vi "VT100translate.vi"(8 "cursor in":i32, 11 "Text":string) -> (0 "cursor out":i32, 3 "Console fixed":string)   [LabVIEW 2021]
panel:
  out "last \\n":i32
  out "string":string
  # "https://vt100.net/docs/vt100-ug/chapter3.html"
  # "http://braun-home.net/michael/info/misc/VT100_commands.htm"
  # "NoneLast login: Mon Aug  2 09:38:15 2021 from 127.0.0.1\n\n\n[1m[7m%[m[1m[0m                                                                               \n \n\n[0m[m[m[Jcrogers@Chriss-Pro ~ % [K[?2004h[?2004l\n\n[1m[7m%[m[1m[0m                                                                               \n \n\n[0m[m[m[Jcrogers@Chriss-Pro ~ % [K[?2004h[?2004l\n\n[1m[7m%[m[1m[0m                                                                               \n \n\n[0m[m[m[Jcrogers@Chriss-Pro ~ % [K[?2004h[?2004l\n\n[1m[7m%[m[1m[0m                                                                               \n \n\n[0m[m[m[Jcrogers@Chriss-Pro ~ % [K[?2004h?2004l\ncrogers@Chriss-Pro ~ % ?2004h?2004l\ncrogers@Chriss-Pro ~ % ?2004h"
  # "ESC [ 13D"
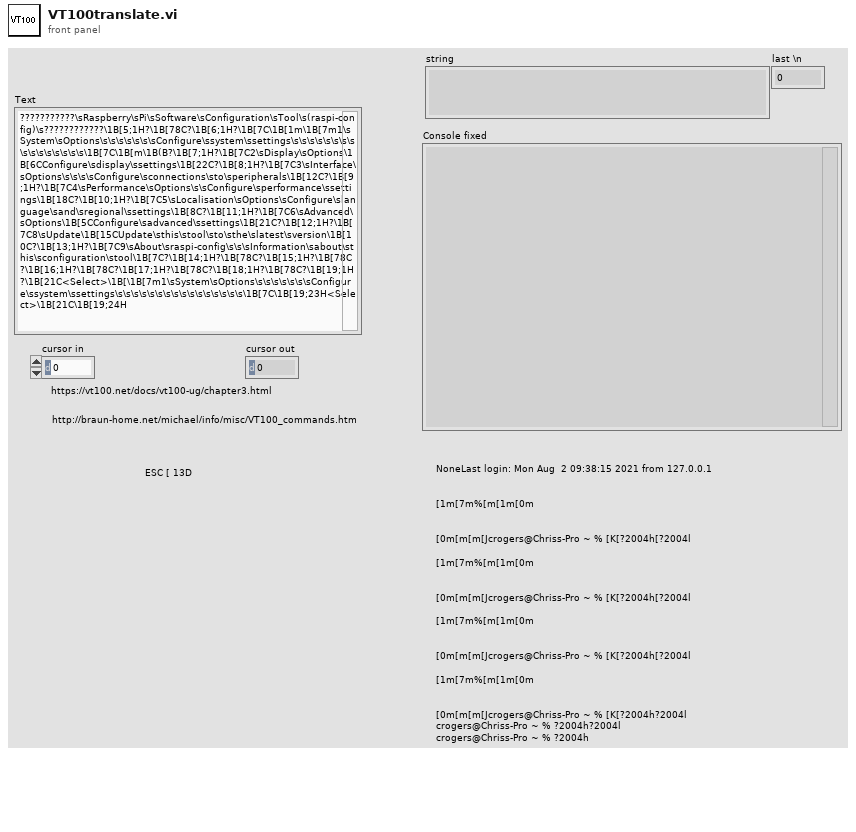
[diagram p1: front panel]
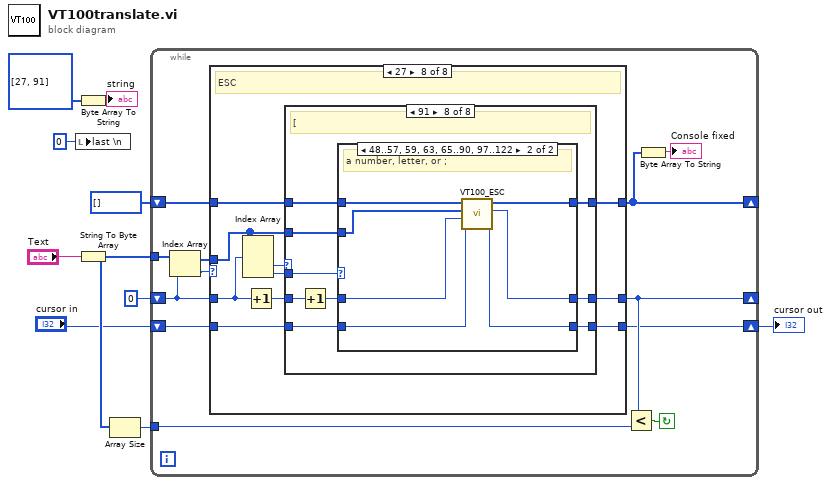
[diagram p0: block diagram]
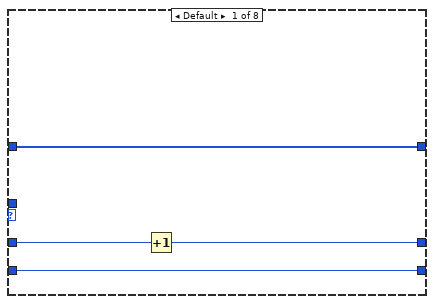
[diagram p2: hidden frame]
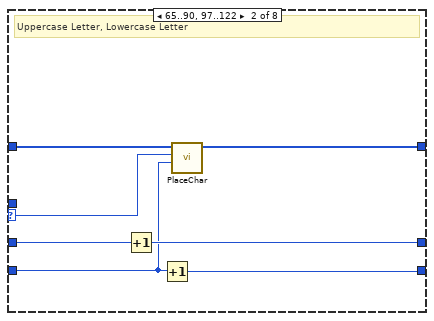
[diagram p3: hidden frame]
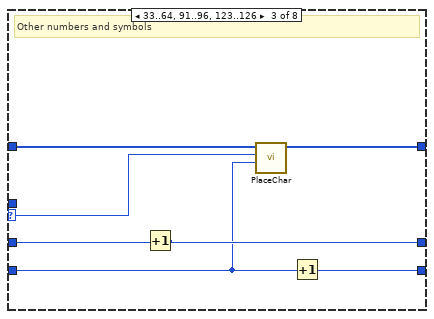
[diagram p4: hidden frame]
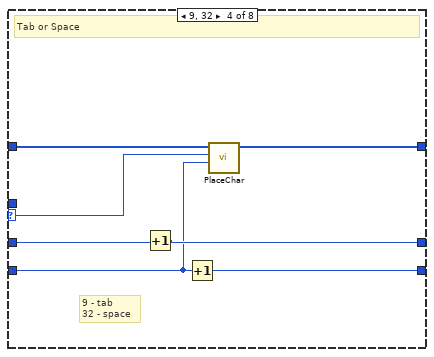
[diagram p5: hidden frame]
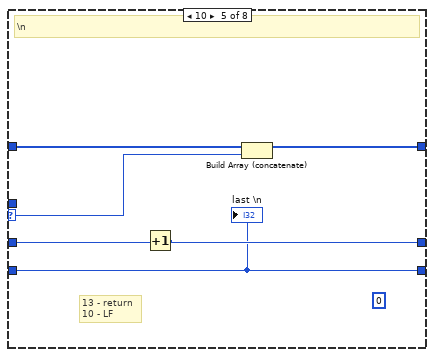
[diagram p6: hidden frame]
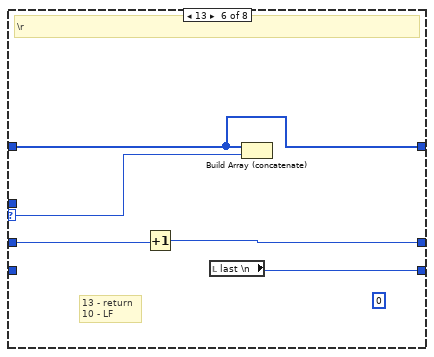
[diagram p7: hidden frame]
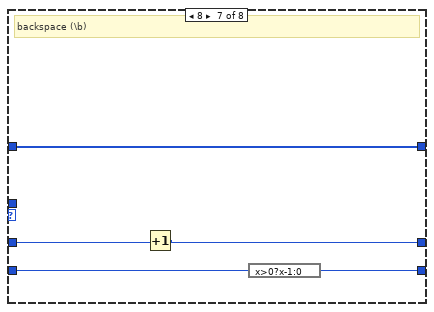
[diagram p8: hidden frame]
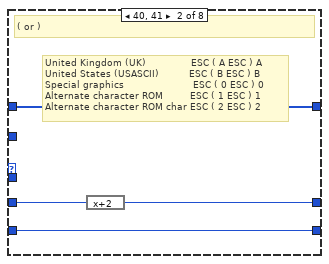
[diagram p10: hidden frame]
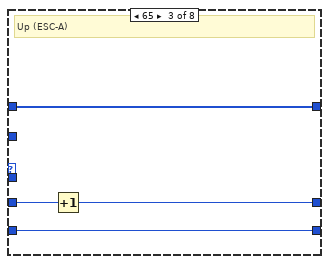
[diagram p11: hidden frame]
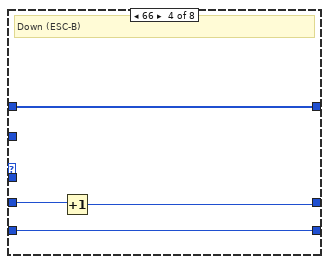
[diagram p12: hidden frame]
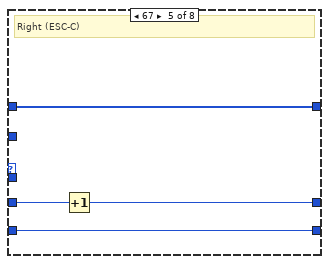
[diagram p13: hidden frame]
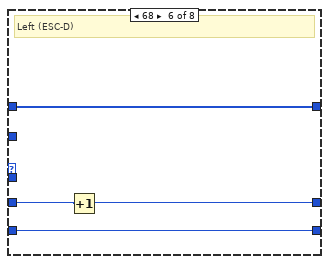
[diagram p14: hidden frame]
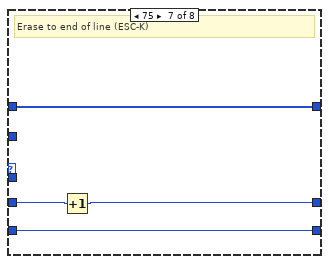
[diagram p15: hidden frame]
diagram:
  n1 = local write "last \\n"(0 ("last \\n")) -> ()
  n2 = Byte Array To String(unsigned byte array=i32[] [27, 91]) -> (string=→"string":string)
  n3 = String To Byte Array(string="Text") -> (unsigned byte array=w9:u8[])
  n4 = Array Size(array=w9) -> (size(s)=w8:i32)
  n5 = while {
    tunnel: w9 -> [w15]
    shift-right: [w17] -> _
    shift-left: 0 -> [w19]
    shift-right: [w12] -> _
    shift-left: u8[] [] -> [w20]
    tunnel: w8 -> [w16]
    shift-right: [w13] -> w5
    shift-left: "cursor in" -> [w14]
    stop <- w18 continue-if-true
    n6 = Index Array(array=w15, index=w19) -> (element=w21:u8)
    n7 = case shown="27" w21 {
      selector: w21 -> [_ w29 w34 w41 w48 w56 _ _]
      tunnel: [w25 w28 w35 w42 w49 w53 w60 w66] -> w12
      tunnel: w20 -> [w25 w27 w36 w43 w50 w53 w60 w67]
      tunnel: w19 -> [w24 w32 w39 w46 w52 w57 w62 w72]
      tunnel: [w23 w31 w38 w45 w51 w55 w61 w69] -> w17
      tunnel: w15 -> [_ _ _ _ _ _ _ w65]
      tunnel: w14 -> [w22 w26 w33 w40 w47 _ w59 w63]
      tunnel: [w22 w30 w37 w44 w47 w54 w58 w64] -> w13
      frame Default {
        n8 = Increment(x=w24) -> (x+1=w23:i32)
      }
      frame 65..90, 97..122 {
        # "Uppercase Letter, Lowercase Letter"
        n9 = Increment(x=w32) -> (x+1=w31:i32)
        n10 = Increment(x=w26) -> (x+1=w30:i32)
        n11 = call "PlaceChar.vi"("cursor in"=w26, "value"=w29, "Array in"=w27) -> ("Array out"=w28:u8[])  [unwired: 8 in]
      }
      frame 33..64, 91..96, 123..126 {
        # "Other numbers and symbols"
        n12 = Increment(x=w39) -> (x+1=w38:i32)
        n13 = call "PlaceChar.vi"("cursor in"=w33, "value"=w34, "Array in"=w36) -> ("Array out"=w35:u8[])  [unwired: 8 in]
        n14 = Increment(x=w33) -> (x+1=w37:i32)
      }
      frame 9, 32 {
        # "9 - tab\n32 - space"
        # "Tab or Space"
        n15 = Increment(x=w46) -> (x+1=w45:i32)
        n16 = Increment(x=w40) -> (x+1=w44:i32)
        n17 = call "PlaceChar.vi"("cursor in"=w40, "value"=w41, "Array in"=w43) -> ("Array out"=w42:u8[])  [unwired: 8 in]
      }
      frame 10 {
        (unwired) 0
        # "13 - return\n10 - LF"
        # "\\n"
        n18 = Increment(x=w52) -> (x+1=w51:i32)
        n19 = Build Array (concatenate)(w50, w48) -> (w49:u8[])
        "last \\n" <- w47
      }
      frame 13 {
        (unwired) 0
        # "13 - return\n10 - LF"
        # "\\r"
        n20 = Increment(x=w57) -> (x+1=w55:i32)
        n21 = local read "last \\n"() -> (w54:i32)
        n22 = Build Array (concatenate)(w53, w56) -> ()  [unwired: 1 out]
      }
      frame 8 {
        # "backspace (\\b)"
        n23 = Increment(x=w62) -> (x+1=w61:i32)
        n24 = expression code="x>0?x-1:0"(w59) -> (w58:i32)
      }
      frame 27 {
        # "ESC"
        n25 = Index Array(array=w65, index #1=w72) -> (element #2=w71:u8, element #3=w68:u8)  [unwired: 2 in, 1 out]
        n26 = Increment(x=w72) -> (x+1=w70:i32)
        n27 = case shown="91" w71 {
          tunnel: w70 -> [w75 w78 w83 w87 w91 w95 w99 w108]
          tunnel: [w75 w77 w82 w86 w90 w94 w98 w105] -> w69
          tunnel: w68 -> [_ _ _ _ _ _ _ w107]
          tunnel: w67 -> [w74 w79 w81 w85 w89 w93 w97 w104]
          tunnel: [w74 w79 w81 w85 w89 w93 w97 w103] -> w66
          tunnel: w65 -> [_ _ _ _ _ _ _ w102]
          tunnel: [w73 w76 w80 w84 w88 w92 w96 w101] -> w64
          tunnel: w63 -> [w73 w76 w80 w84 w88 w92 w96 w100]
          frame Default {
          }
          frame 40, 41 {
            # "United Kingdom (UK)\t              ESC ( A\tESC ) A\nUnited States (USASCII)\t         ESC ( B\tESC ) B\nSpecial graphics \t                     ESC ( 0\tESC ) 0\nAlternate character ROM\t        ESC ( 1\tESC ) 1\nAlternate character ROM char\tESC ( 2\tESC ) 2"
            # "( or )"
            n28 = expression code="x+2"(w78) -> (w77:i32)
          }
          frame 65 {
            # "Up (ESC-A)"
            n29 = Increment(x=w83) -> (x+1=w82:i32)
          }
          frame 66 {
            # "Down (ESC-B)"
            n30 = Increment(x=w87) -> (x+1=w86:i32)
          }
          frame 67 {
            # "Right (ESC-C)"
            n31 = Increment(x=w91) -> (x+1=w90:i32)
          }
          frame 68 {
            # "Left (ESC-D)"
            n32 = Increment(x=w95) -> (x+1=w94:i32)
          }
          frame 75 {
            # "Erase to end of line (ESC-K)"
            n33 = Increment(x=w99) -> (x+1=w98:i32)
          }
          frame 91 {
            # "["
            n34 = Increment(x=w108) -> (x+1=w106:i32)
            n35 = case shown="48..57, 59, 63, 65..90, 97..122" w107 {
              tunnel: w106 -> [w111 w115]
              tunnel: [w111 w114] -> w105
              tunnel: w104 -> [w110 w117]
              tunnel: [w110 w116] -> w103
              tunnel: w102 -> [_ w118]
              tunnel: [w109 w112] -> w101
              tunnel: w100 -> [w109 w113]
              frame Default {
              }
              frame 48..57, 59, 63, 65..90, 97..122 {
                # "a number, letter, or ;"
                n36 = call "VT100_ESC.vi"("cursor in"=w113, "index in"=w115, "Original data"=w118, "Data in"=w117) -> ("cursor out"=w112:i32, "index out"=w114:i32, "Data out"=w116:u8[])  [unwired: 5 in]
              }
            }
          }
        }
      }
    }
    n37 = Less?(x=w17, y=w16) -> (x < y?=w18:bool)
    n38 = Byte Array To String(unsigned byte array=w12) -> (string=→"Console fixed":string)
  }
  "cursor out" <- w5
